vi "Calculate Sweep Timeout.vi"(0 "VISA resource name":refnum<visa-resource-name>, 1 "Voltage Sweep Start (0V)":dbl, 2 "Voltage Sweep Stop (10V)":dbl=10.0, 3 "Voltage Sweep Step Size (1V)":dbl=1.0, 5 "Voltage Sweep Delay (1s)":dbl=1.0, 11 "error in (no error)":errorcluster) -> (4 "VISA resource name out":refnum<visa-resource-name>, 6 "Steps":dbl, 15 "error out":errorcluster)   [LabVIEW 2021, in "Keithley 648X Series.lvlib"]
doc: "This private VI works in tandem with <b>Set Sweep Timeout</b> to control the VISA timeout settings. This is necessary due to the instrument not responding to queries in a timely manner when performing a voltage sweep."
uses:
  <instrlib>/Keithley 648X Series/Keithley 648X Series.lvlib
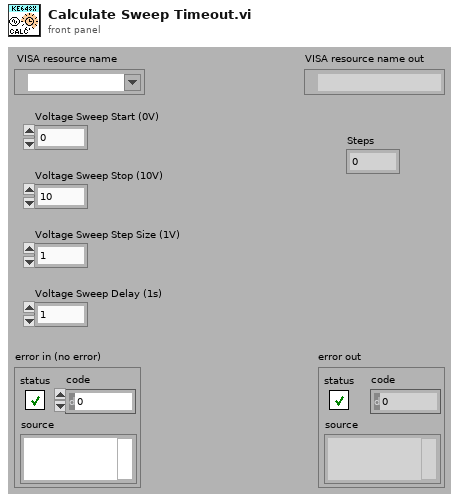
[diagram p1: front panel]
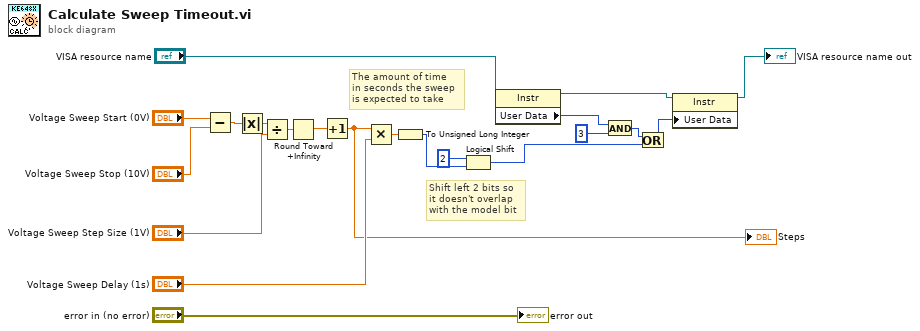
[diagram p0: block diagram]
diagram:
  # "Shift left 2 bits so\nit doesn't overlap \nwith the model bit"
  # "The amount of time\nin seconds the sweep\nis expected to take"
  n1 = Subtract(x="Voltage Sweep Start (0V)", y="Voltage Sweep Stop (10V)") -> (x-y=w18:dbl)
  n2 = Absolute Value(x=w18) -> (abs(x)=w17:dbl)
  n3 = Divide(x=w17, y="Voltage Sweep Step Size (1V)") -> (x/y=w3:dbl)
  n4 = Round Toward +Infinity(x=w3) -> (ceil(x): smallest int >= x=w2:dbl)
  n5 = Increment(x=w2) -> (x+1=w1:dbl)
  "Steps" <- w1
  n6 = Multiply(x=w1, y="Voltage Sweep Delay (1s)") -> (x*y=w14:dbl)
  n7 = To Unsigned Long Integer(number=w14) -> (unsigned 32bit integer=w13:u32)
  n8 = Logical Shift(y=i16 2, x=w13) -> (x << y=w8:u32)
  n9 = property class="Instr"(reference="VISA resource name") -> (reference out=w7:refnum<visa-resource-name>, "User Data"=w10:u32)  [unwired: 1 in, 1 out]
  n10 = And(x=w10, y=u32 3) -> (x .and. y?=w9:u32)
  n11 = Or(x=w9, y=w8) -> (x .or. y?=w4:u32)
  n12 = property class="Instr"(reference=w7, "User Data"=w4) -> (reference out=→"VISA resource name out":refnum<visa-resource-name>)  [unwired: 1 in, 1 out]
  "error out" <- "error in (no error)"
